vi "Get Window Name.vi"(8 "error in":errorcluster caption="error in (no error)" {"code" format="%d\n%x"}, 11 "window refnum in":T1 caption="window refnum in (NaWR)") -> (0 "error out":errorcluster {"code" format="%d\n%x"}, 2 "window name":string, 3 "window refnum out":T1)   [LabVIEW 2020, in "Win Util New.lvlib"]
doc: "This VI will use window refnum in to get the name of a window. The name of a window is simply the text appearing in the title bar of the window. If the title bar of the window is not shown, the name of the window will be a NULL string."
uses:
  Win Util New.lvlib
  Window Refnum.ctl
  user32.dll
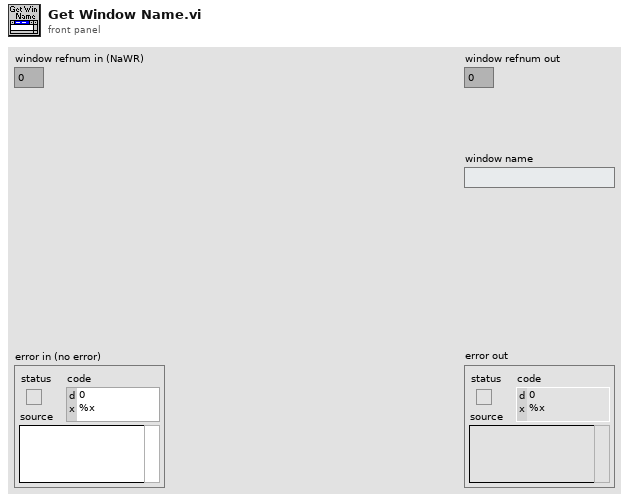
[diagram p1: front panel]
types:
  T1 = typedef "Win Util New.lvlib/Window Refnum.ctl" = u64
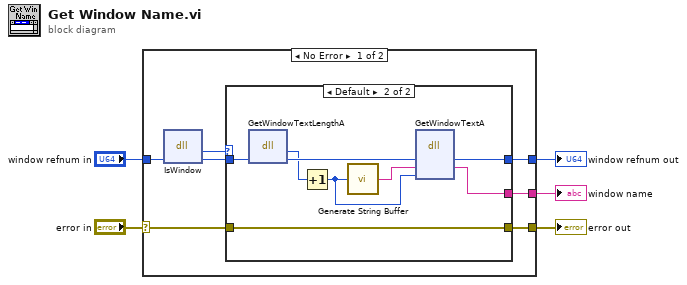
[diagram p0: block diagram]
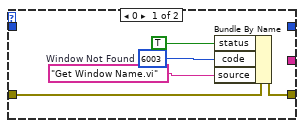
[diagram p2: hidden frame]
diagram:
  n1 = case shown="No Error" "error in" {
    selector: "error in" -> [w11 w27]
    tunnel: "window refnum in" -> [w12 w26]
    tunnel: [w10 w27] -> w3
    tunnel: [w7 _] -> w4
    tunnel: [w6 w26] -> w1
    frame No Error {
      n2 = dll-call lib="user32.dll" fn="IsWindow"("hWnd"=w12) -> ("IsWindow?"=w9:i32, "hWnd"=w8:u64)  [unwired: 3 in, 2 out]
      n3 = case shown="Default" w9 {
        tunnel: w11 -> [w14 w22]
        tunnel: [w17 w22] -> w10
        tunnel: w8 -> [_ w23]
        tunnel: [_ w21] -> w7
        tunnel: [_ w20] -> w6
        frame 0 {
          w16 = 6003  # Window Not Found
          n4 = Bundle By Name(cluster=w14, "status"=TRUE ("show call chain? (False)"), "code"=w16, "source"="Get Window Name.vi") -> (w17:errorcluster)
        }
        frame Default {
          n5 = dll-call lib="user32.dll" fn="GetWindowTextLengthA" label="GetWindowTextLength"("hWnd"=w23) -> ("length"=w19:i32, "hWnd"=w24:u64)  [unwired: 3 in, 2 out]
          n6 = Increment(x=w19) -> (x+1=w18:i32)
          n7 = call "Generate String Buffer.vi"("buffer size"=w18) -> ("string buffer"=w25:string)
          n8 = dll-call lib="user32.dll" fn="GetWindowTextA" label="GetWindowText"("hWnd"=w24, "NameBuffer"=w25, "MaxCharsToCopy"=w18) -> ("hWnd"=w20:u64, "NameBuffer"=w21:string)  [unwired: 4 in, 3 out]
        }
      }
    }
    frame Error {
    }
  }
  "error out" <- w3
  "window name" <- w4
  "window refnum out" <- w1
